vi "Unflatten Value.vi"(8 "error in (no error)":errorcluster, 10 "Value":string, 11 "Boolean in":refnum<class "Timestamp.lvclass">) -> (0 "error out":errorcluster, 3 "Boolean out":refnum<class "Timestamp.lvclass">)   [LabVIEW 2017, in "Timestamp.lvclass"]
uses:
  <vilib>/gpm_packages/@cs/data-type-serializer/source/Timestamp/Timestamp.lvclass
  <vilib>/gpm_packages/@cs/data-type-serializer/source/Timestamp/Timestamp.lvclass/Timestamp.ctl
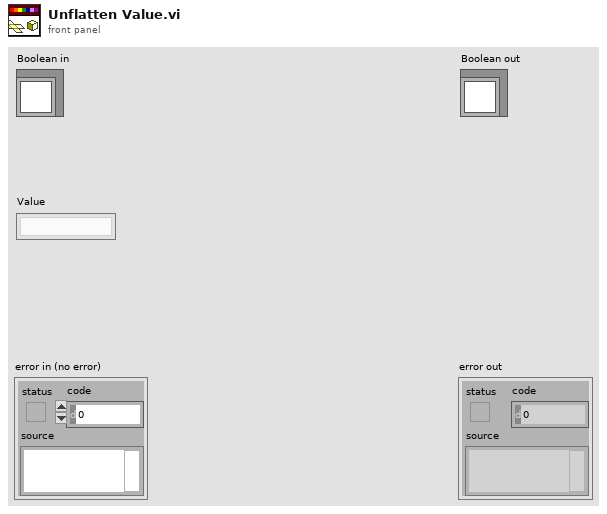
[diagram p1: front panel]
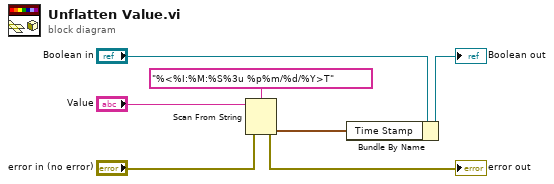
[diagram p0: block diagram]
diagram:
  n1 = Scan From String(format string="%<%I:%M:%S%3u %p%m/%d/%Y>T", input string="Value", error in="error in (no error)") -> (error out=→"error out":errorcluster, output 1=w3:timestamp)  [unwired: 2 in, 2 out]
  n2 = Bundle By Name(cluster="Boolean in", "Time Stamp"=w3) -> (→"Boolean out":refnum<class "Timestamp.lvclass">)
